vi "SubVI_DisplayBestResults.vi"(1 "Dissimilarity values (in)":dbl[](array[numeric]), 2 "Objects to compare it to":string[](array[string]), 3 "Check also circle":bool) -> (0 "Result":string)   [LabVIEW 2018]
panel:
  out "min index(es)":i32
  out "Dissimilarity values":dbl[](array[numeric])
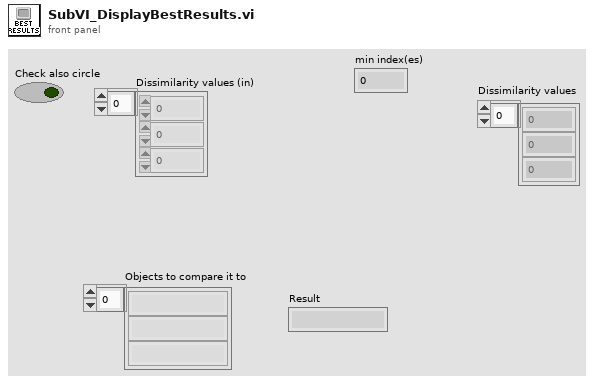
[diagram p1: front panel]
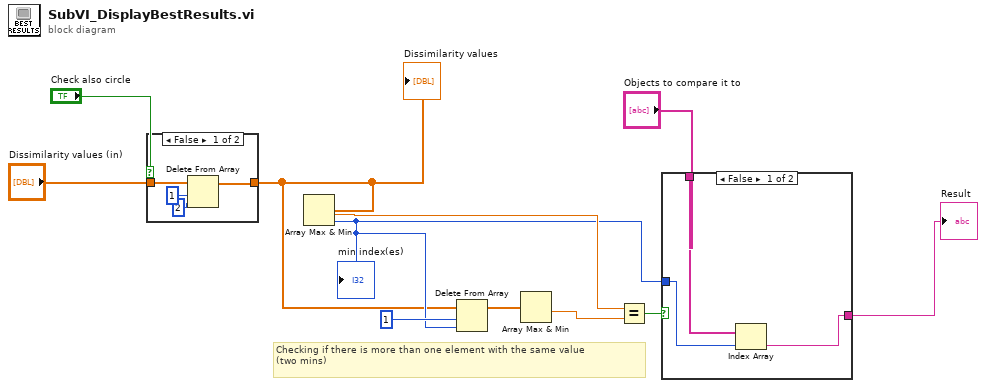
[diagram p0: block diagram]
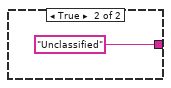
[diagram p3: hidden frame]
diagram:
  # "Checking if there is more than one element with the same value\n(two mins)"
  n1 = case shown="False" "Check also circle" {
    tunnel: "Dissimilarity values (in)" -> [w15 w16]
    tunnel: [w12 w16] -> w2
    frame False {
      n2 = Delete From Array(array=w15, length=1, index=2) -> (array with subset deleted=w12:dbl[])  [unwired: 1 out]
    }
    frame True {
    }
  }
  "Dissimilarity values" <- w2
  n3 = Array Max & Min(array=w2) -> (min value=w8:dbl, min index (indices)=w5:i32)  [unwired: 2 out]
  "min index(es)" <- w5
  n4 = Delete From Array(array=w2, length=1, index=w5) -> (array with subset deleted=w9:dbl[])  [unwired: 1 out]
  n5 = Array Max & Min(array=w9) -> (min value=w7:dbl)  [unwired: 3 out]
  n6 = Equal?(x=w8, y=w7) -> (x = y?=w10:bool)
  n7 = case shown="False" w10 {
    tunnel: [w17 "Unclassified"] -> w6
    tunnel: w5 -> [w18 _]
    tunnel: "Objects to compare it to" -> [w19 _]
    frame False {
      n8 = Index Array(array=w19, index=w18) -> (element=w17:string)
    }
    frame True {
    }
  }
  "Result" <- w6
